vi "SVM_Calculator.vi"(5 "ERP_all_icon":dbl[][](array[numeric]) format="%0.3f", 7 "ModelFileName":string="C:\\\\WORK\\\\RBFModel", 8 "Target_total2 (from offline file)":path=path "C:/Users/Jaehong/Desktop/안전복지프로젝트/LabVIEW/RSVP_offline_onine/분석데이터/전선미_RSVP_Offline_Analysis2/2014-09-01/Target_Total2.txt", 11 "ERP_Parameters_of_Target_prior.txt":path=path "C:/Users/Jaehong/Desktop/안전복지프로젝트/LabVIEW/RSVP_offline_onine/분석데이터/전선미_RSVP_Training_Test(LDA)/2014-08-29/ERP_Parameters_of_Target_prior.txt") -> (1 "ACC1(%)":dbl, 3 "Accuracy2(%)":dbl)   [LabVIEW 2013]
uses:
  <vilib>/Utility/file.llb/Read From Spreadsheet File (I64).vi
  <vilib>/Utility/file.llb/Read From Spreadsheet File (DBL).vi
panel:
  out "size(s)":i32[](array[numeric])
  out "selected_all":i16[](array[numeric])
  out "test predict":dbl[](array[numeric])=[-1.0, -1.0, -1.0, -1.0, -1.0, -1.0, -1.0, -1.0, -1.0, -1.0, -1.0, -1.0, -1.0, -1.0, -1.0, -1.0, -1.0, -1.0, -1.0, -1.0, -1.0, -1.0, -1.0, -1.0, 1.0, -1.0, 1.0, 1.0, -1.0, 1.0, -1.0, -1.0, -1.0, -1.0, -1.0, -1.0, 1.0, -1.0, 1.0, -1.0, 1.0, -1.0, -1.0, -1.0]
  out "Squared correlation\n coefficient":dbl
  out "Total":i32
  out "correct":i16
  # "Results"
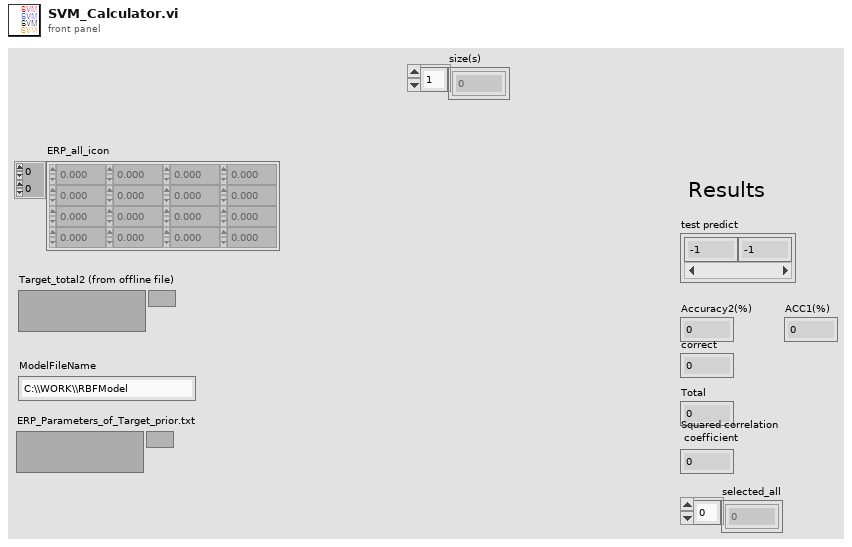
[diagram p1: front panel]
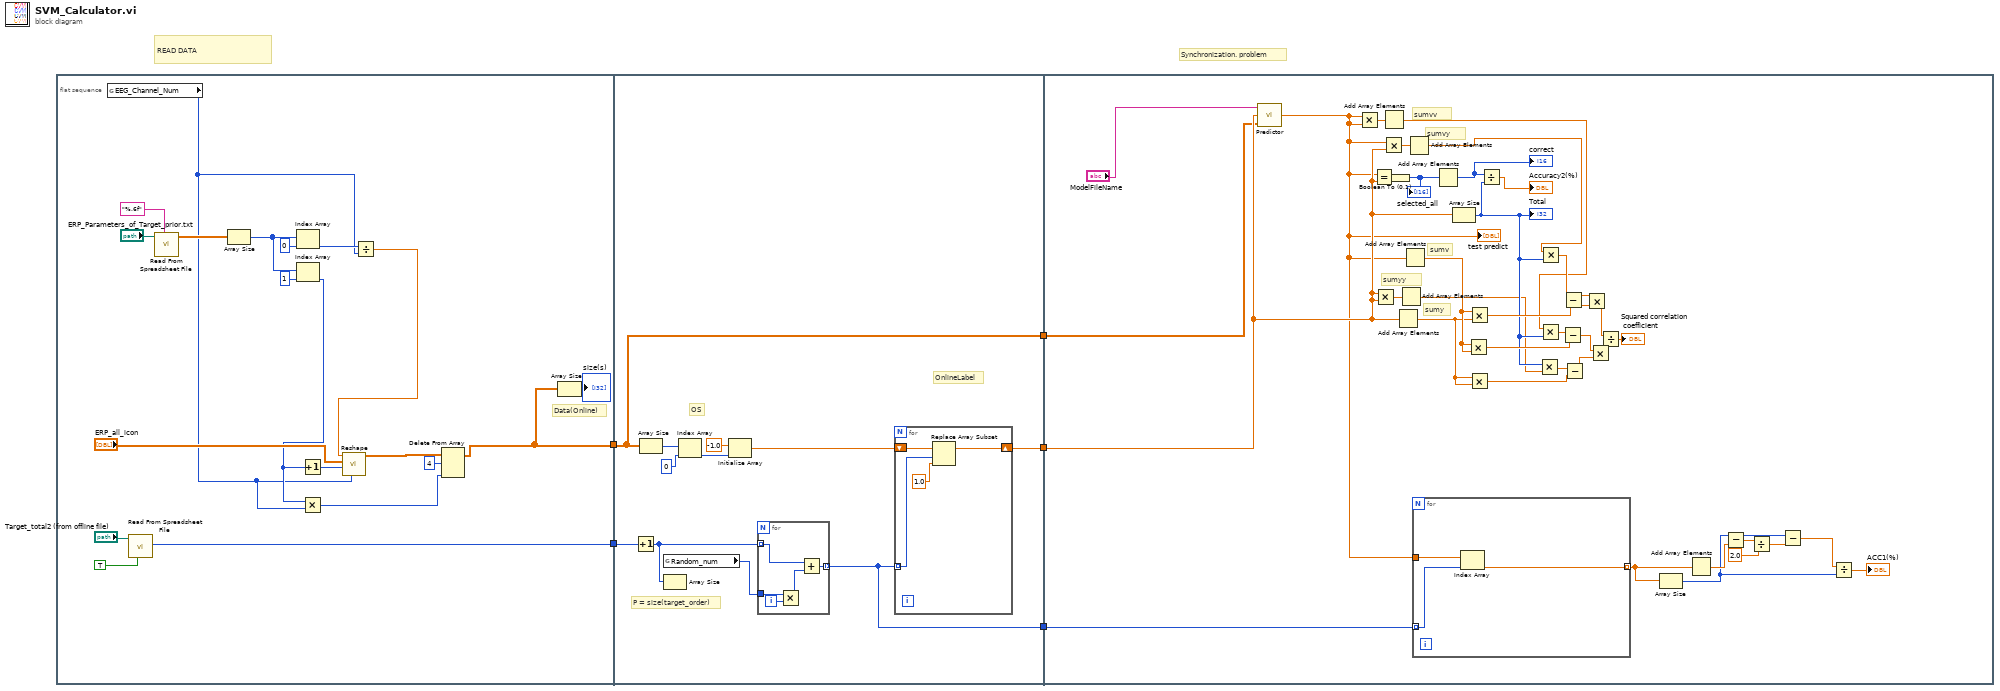
[diagram p0: block diagram]
diagram:
  # "Synchronization. problem"
  # "READ DATA"
  n1 = flat-sequence {
    tunnel: [w8] -> w5
    tunnel: [w23] -> w4
    tunnel: w5 -> [w27]
    tunnel: w4 -> [w34]
    tunnel: [w28] -> w3
    tunnel: [w27] -> w2
    tunnel: [w26] -> w1
    tunnel: w3 -> [w58]
    tunnel: w2 -> [w46]
    tunnel: w1 -> [w57]
    frame #0 {
      # "Data(Online)"
      n2 = global read "Control_Panel.vi" "EEG_Channel_Num"() -> (w6:i32)
      n3 = call-poly <vilib>:"Read From Spreadsheet File.vi"("transpose (no:F)"=TRUE, "file path (dialog if empty)"="Target_total2 (from offline file)") -> ("first row"=w23:i64[])  [unwired: 5 in, 4 out]
      n4 = call-poly <vilib>:"Read From Spreadsheet File.vi"("format (%.3f)"="%.6f", "file path (dialog if empty)"="ERP_Parameters_of_Target_prior.txt") -> ("all rows"=w17:dbl[][])  [unwired: 5 in, 4 out]
      n5 = Array Size(array=w17) -> (size(s)=w20:i32[])
      n6 = Index Array(array=w20, index=0) -> (element=w21:i32)
      n7 = Index Array(array=w20, index=1) -> (element=w7:i32)
      n8 = Increment(x=w7) -> (x+1=w11:i32)
      n9 = Multiply(x=w7, y=w6) -> (x*y=w13:i32)
      n10 = Divide(x=w21, y=w6) -> (x/y=w10:dbl)
      n11 = call "Reshape.vi"("Numeric"=w6, "EEG_Channel_Num"=w11, "all rows"="ERP_all_icon", "Numeric 2"=w10) -> ("Array"=w14:dbl[][])  [unwired: 7 in]
      n12 = Delete From Array(array=w14, length=4, index (col)=w13) -> (array with subset deleted=w8:dbl[][])  [unwired: 1 in, 1 out]
      n13 = Array Size(array=w8) -> (size(s)=→"size(s)":i32[])
    }
    frame #1 {
      # "OnlineLabel"
      # "P = size(target_order)"
      # "OS"
      n14 = Increment(x=w34) -> (x+1=w33:i64[])
      n15 = Array Size(array=w27) -> (size(s)=w36:i32[])
      n16 = global read "Control_Panel.vi" "Random_num"() -> (w32:i32)
      n17 = Array Size(array=w33) -> ()  [unwired: 1 out]
      n18 = Index Array(array=w36, index=0) -> (element=w31:i32)
      n19 = Initialize Array(-1.0 ("element"), w31) -> (w29:dbl[])
      n20 = for {
        tunnel: w33 -> [w42] mode=indexing
        tunnel: w32 -> [w44]
        tunnel: [w41] -> w26 mode=indexing
        i -> [w45]
        n21 = Multiply(x=w44, y=w45) -> (x*y=w43:i32)
        n22 = Add(x=w42, y=w43) -> (x+y=w41:i64)
      }
      n23 = for {
        tunnel: w26 -> [w39] mode=indexing
        shift-right: [w37] -> w28
        shift-left: w29 -> [w40]
        n24 = Replace Array Subset(array=w40, new element=1.0 ("new element/subarray"), index=w39) -> (w37:dbl[])
      }
    }
    frame #2 {
      # "sumyy"
      # "sumvy"
      # "sumvv"
      # "sumy"
      # "sumv"
      n25 = call "Predictor.vi"("attributes"=w46, "Lables"=w58, "ModelFileName"="ModelFileName") -> ("predictedlevel"=w56:dbl[])
      "test predict" <- w56
      n26 = Multiply(x=w56, y=w56) -> (x*y=w66:dbl[])
      n27 = Equal?(x=w56, y=w58) -> (x = y?=w61:bool[])
      n28 = Multiply(x=w58, y=w58) -> (x*y=w65:dbl[])
      n29 = Multiply(x=w56, y=w58) -> (x*y=w67:dbl[])
      n30 = Add Array Elements(numeric array=w66) -> (sum=w63:dbl)
      n31 = Boolean To (0,1)(Boolean=w61) -> (0, 1=w62:i16[])
      "selected_all" <- w62
      n32 = Add Array Elements(numeric array=w58) -> (sum=w75:dbl)
      n33 = Add Array Elements(numeric array=w65) -> (sum=w60:dbl)
      n34 = Add Array Elements(numeric array=w56) -> (sum=w78:dbl)
      n35 = Add Array Elements(numeric array=w67) -> (sum=w64:dbl)
      n36 = for {
        tunnel: w57 -> [w85] mode=indexing
        tunnel: w56 -> [w86]
        tunnel: [w84] -> w55 mode=indexing
        n37 = Index Array(array=w86, index=w85) -> (element=w84:dbl)
      }
      n38 = Add Array Elements(numeric array=w62) -> (sum=w59:i16)
      "correct" <- w59
      n39 = Array Size(array=w58) -> (size(s)=w68:i32)
      "Total" <- w68
      n40 = Multiply(x=w78, y=w78) -> (x*y=w77:dbl)
      n41 = Multiply(x=w78, y=w75) -> (x*y=w81:dbl)
      n42 = Multiply(x=w75, y=w75) -> (x*y=w74:dbl)
      n43 = Divide(x=w59, y=w68) -> (x/y=→"Accuracy2(%)":dbl)
      n44 = Multiply(x=w68, y=w60) -> (x*y=w76:dbl)
      n45 = Multiply(x=w63, y=w68) -> (x*y=w79:dbl)
      n46 = Multiply(x=w64, y=w68) -> (x*y=w82:dbl)
      n47 = Subtract(x=w79, y=w77) -> (x-y=w73:dbl)
      n48 = Subtract(x=w82, y=w81) -> (x-y=w80:dbl)
      n49 = Subtract(x=w76, y=w74) -> (x-y=w72:dbl)
      n50 = Multiply(x=w80, y=w80) -> (x*y=w71:dbl)
      n51 = Multiply(x=w73, y=w72) -> (x*y=w70:dbl)
      n52 = Divide(x=w71, y=w70) -> (x/y=→"Squared correlation\n coefficient":dbl)
      n53 = Array Size(array=w55) -> (size(s)=w48:i32)
      n54 = Add Array Elements(numeric array=w55) -> (sum=w52:dbl)
      n55 = Subtract(x=w48, y=w52) -> (x-y=w51:dbl)
      n56 = Divide(x=w51, y=2.0) -> (x/y=w49:dbl)
      n57 = Subtract(x=w48, y=w49) -> (x-y=w47:dbl)
      n58 = Divide(x=w47, y=w48) -> (x/y=→"ACC1(%)":dbl)
    }
  }
